vi "ChangeModDate_SingleFile.vi"(8 "error in (no error)":errorcluster, 11 "appended path":path) -> (0 "error out":errorcluster, 1 "element":string, 2 "output 1":timestamp)   [LabVIEW 2015, in "EMG.lvclass"]
uses:
  EMG.lvclass
  CustomVIs/CustomVI.lvlib
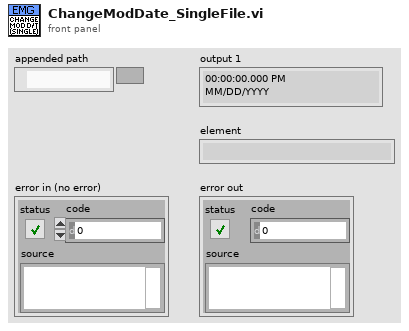
[diagram p1: front panel]
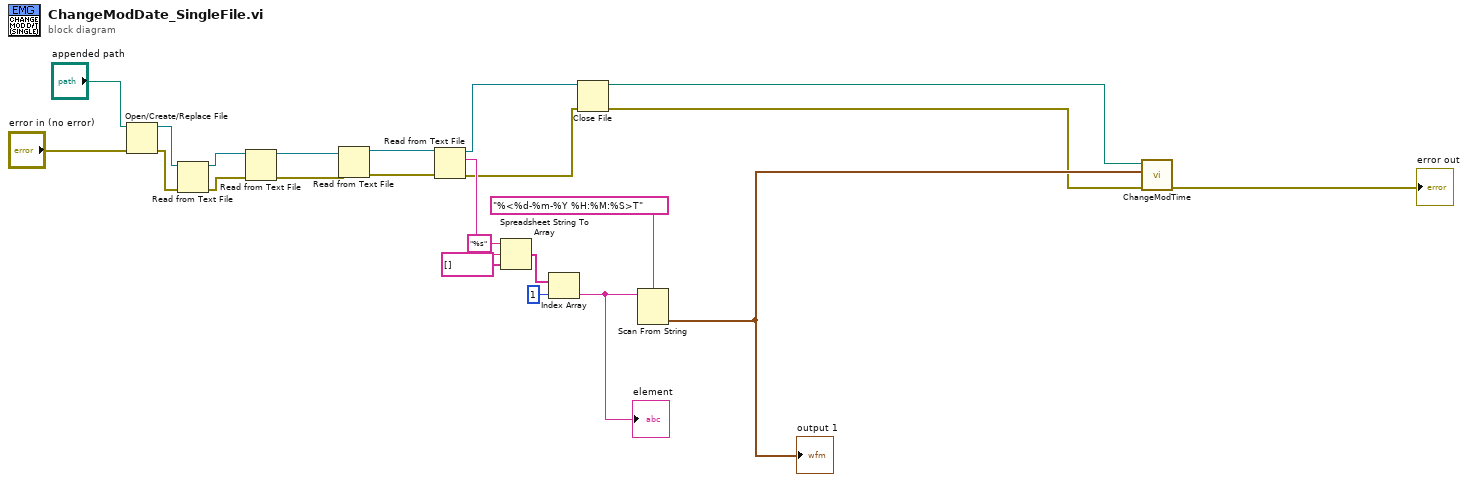
[diagram p0: block diagram]
diagram:
  n1 = Open/Create/Replace File(file path (use dialog)="appended path", error in="error in (no error)") -> (refnum out=w1:refnum<file>, error out=w2:errorcluster)  [unwired: 4 in, 1 out]
  n2 = Read from Text File(file (use dialog)=w1, error in=w2) -> (refnum out=w3:refnum<file>, error out=w4:errorcluster)  [unwired: 2 in, 2 out]
  n3 = Read from Text File(file (use dialog)=w3, error in=w4) -> (refnum out=w5:refnum<file>, error out=w6:errorcluster)  [unwired: 2 in, 2 out]
  n4 = Read from Text File(file (use dialog)=w5, error in=w6) -> (refnum out=w7:refnum<file>, error out=w8:errorcluster)  [unwired: 2 in, 2 out]
  n5 = Read from Text File(file (use dialog)=w7, error in=w8) -> (refnum out=w10:refnum<file>, text=w13:string, error out=w9:errorcluster)  [unwired: 2 in, 1 out]
  n6 = Spreadsheet String To Array(format string="%s", spreadsheet string=w13, array type (2D Dbl)=string[] []) -> (array=w16:string[])  [unwired: 1 in]
  n7 = Index Array(array=w16, index=1) -> (element=w18:string)
  "element" <- w18
  n8 = Close File(refnum=w10, error in=w9) -> (path=w12:path, error out=w11:errorcluster)
  n9 = Scan From String(format string="%<%d-%m-%Y %H:%M:%S>T", input string=w18) -> (output 1=w20:timestamp)  [unwired: 3 in, 3 out]
  "output 1" <- w20
  n10 = call "ChangeModTime.vi"("error in (no error)"=w11, "Time Stamp"=w20, "path"=w12) -> ("error out"=→"error out":errorcluster)  [unwired: 7 in, 1 out]
